vi "SQLite Edit Balance Test.vi"(8 "Error In (no error)":errorcluster) -> (0 "Error Out":errorcluster)   [LabVIEW 2023]
uses:
  <vilib>/addons/_JKI Toolkits/Caraya/classes/Test/Test.lvclass
  Clasess/SQLite DB Operator/SQLite DB Operator.lvclass
  <vilib>/drjdpowell/SQLite Library/SQLite.lvlib
  <vilib>/addons/_JKI Toolkits/Caraya/classes/Assert/Assert.lvclass
  <vilib>/drjdpowell/SQLite Library/SQL Connection/Execute SQL (No results).vi
  <vilib>/drjdpowell/SQLite Library/SQL Connection/Connection.lvclass
  <vilib>/addons/_JKI Toolkits/Caraya/classes/Assert/Assert Not Equal Value_Variant.vi
  <vilib>/addons/_JKI Toolkits/Caraya/classes/Assert/Assert Equal Value_Variant.vi
  <vilib>/drjdpowell/SQLite Library/SQL Connection/Execute SQL (Variant Cluster results).vi
  H:/Desktop/LabVIEW/LabView Repo/Expenses-Tracker-DB-Operator/SQLite DB Operator/SQLite DB Operator.lvclass
  H:/Desktop/LabVIEW/LabView Repo/Expenses-Tracker-DB-Operator/Database Interactions/Database Interactions.lvclass
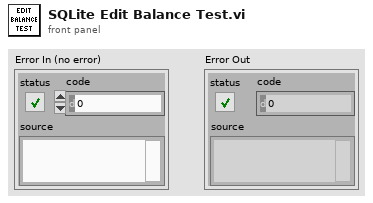
[diagram p1: front panel]
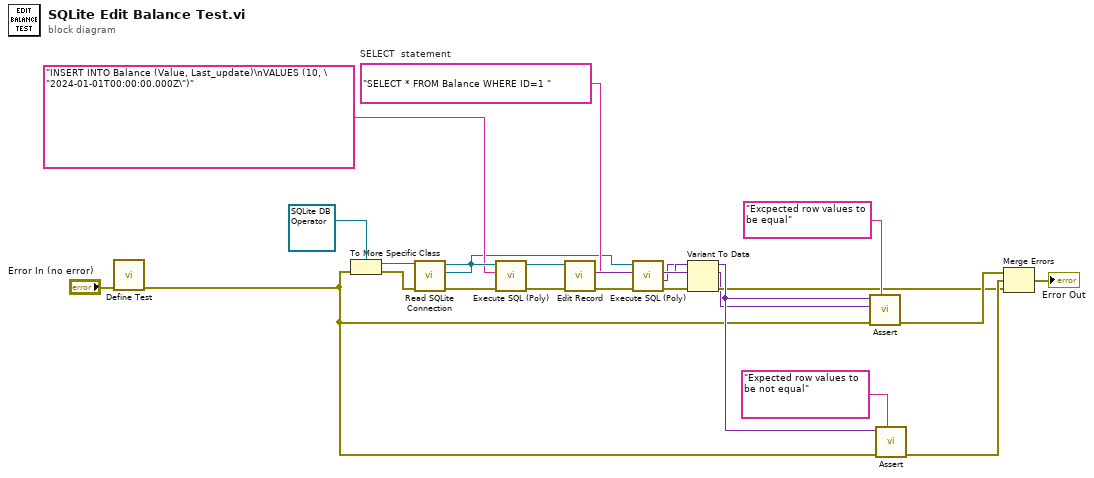
[diagram p0: block diagram]
diagram:
  w6 = "SELECT * FROM Balance WHERE ID=1 "  # SELECT  statement
  n1 = call <vilib>:"Define Test.vi"("error in (no error)"="Error In (no error)") -> ("error out"=w13:errorcluster)  [unwired: 9 in, 1 out]
  n2 = To More Specific Class(target class=refnum<class "SQLite DB Operator.lvclass"> refnum ("SQLite DB Operator.lvclass"), error in=w13) -> (reference=w12:refnum<vi>, specific class reference=w25:refnum<class "SQLite DB Operator.lvclass">, error out=w19:errorcluster)
  n3 = call "Read SQLite Connection.vi"("Error In (no error)"=w19, "SQLite DB Operator In"=w25) -> ("Error Out"=w23:errorcluster, "SQLite.lvlib:Connection"=w5:refnum<class "Connection.lvclass">, "SQLite DB Operator out"=w10:refnum<class "SQLite DB Operator.lvclass">)  [unwired: 7 in]
  n4 = call-poly <vilib>:"Execute SQL (Poly).vi"("error in (no error)"=w23, "SQL"="INSERT INTO Balance (Value, Last_update)\nVALUES (10, \"2024-01-01T00:00:00.000Z\")", "SQLite Connection in"=w5) -> ("error out"=w11:errorcluster)  [unwired: 7 in, 1 out]
  n5 = call-dynamic "Edit Record.vi"("Error In (no error)"=w11, 10:w9, "SQLite DB Operator In"=w10) -> ("Error Out"=w7:errorcluster)  [unwired: 7 in, 1 out]
  n6 = call-poly <vilib>:"Execute SQL (Poly).vi"("error in (no error)"=w7, "SQL"=w6, "SQLite Connection in"=w5) -> ("error out"=w3:errorcluster, "Result (use Variant to Data)"=w4:variant, "Cluster"=w1:variant)  [unwired: 5 in, 1 out]
  n7 = Variant To Data(error in=w3, type=w1, Variant=w4) -> (data=w17:variant, error out=w14:errorcluster)
  n8 = call-poly <vilib>:"Assert.vi"("Label"="Excpected row values to be equal" ("Label (VI Title)"), "error in (no error)"=w13, "X"=w17) -> ("error out"=w20:errorcluster, "Y"=w9:variant)  [unwired: 6 in, 1 out]
  n9 = call-poly <vilib>:"Assert.vi"("Label"="Expected row values to be not equal" ("Label (VI Title)"), "error in (no error)"=w13, "X"=w17) -> ("error out"=w15:errorcluster, "Y"=w2:variant)  [unwired: 6 in, 1 out]
  n10 = Merge Errors(w20, w15, w14) -> (→"Error Out":errorcluster)
